vi "Measurement Logic.vi"() -> ()   [LabVIEW 2021, in "Quiescent Current_PMIC.lvlib"]
uses:
  Quiescent Current_PMIC.lvlib
  <instrlib>/niDCPower/nidcpower.llb/niDCPower Source Mode.ctl
  <instrlib>/niDCPower/nidcpower.llb/niDCPower Wait For Event - Event.ctl
  <instrlib>/niDCPower/nidcpower.llb/niDCPower Get Channel Name From String.vi
  <instrlib>/niDCPower/nidcpower.llb/niDCPower Output Function.ctl
  <instrlib>/niDCPower/nidcpower.llb/niDCPower Sequence Attribute Type.ctl
  <instrlib>/niDCPower/nidcpower.llb/niDCPower Create Advanced Sequence Step With Channels.vi
  Measurement Results.ctl
  <vilib>/Plug-In SDKs/Measurements/Measure Call Context/Measure Call Context.lvclass
  Measurement Configuration.ctl
panel:
  out "measurement results":T1
  in  "measurement configuration":T2={"DUT setup time"=1.0, "Source delay"=0.005, "Aperture time"=0.005, "Source resource name"="", "Source sense"=0, "Source current limit"=25.0, "Source maximum power"=300.0, "Source start voltage"=6.0, "Source stop voltage"=20.0, "Source voltage sweep points"=10} {"Source sense" items=["Local"=1008, "Remote"=1009]}
  out "measure call context out":refnum<class "Measure Call Context.lvclass">
  in  "measure call context in":refnum<class "Measure Call Context.lvclass">
  out "error out":errorcluster
  in  "error in":errorcluster
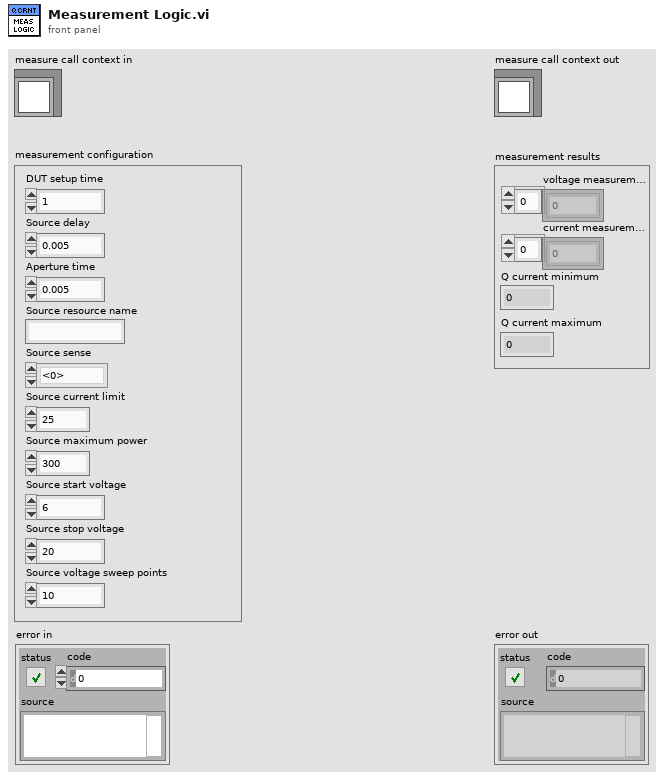
[diagram p1: front panel]
types:
  T1 = typedef "Quiescent Current_PMIC.lvlib/Measurement Results.ctl" = cluster{"Source voltages":dbl[], "Q currents":dbl[], "Q current minimum":dbl, "Q current maximum":dbl}
  T2 = typedef "Quiescent Current_PMIC.lvlib/Measurement Configuration.ctl" = cluster{"DUT setup time":dbl, "Source delay":dbl, "Aperture time":dbl, "Source resource name":string, "Source sense":i32, "Source current limit":dbl, "Source maximum power":dbl, "Source start voltage":dbl, "Source stop voltage":dbl, "Source voltage sweep points":i32}
  T3 = typedef "niDCPower Wait For Event - Event.ctl" = i32
  T4 = typedef "niDCPower Sequence Attribute Type.ctl" = i32
  T5 = typedef "niDCPower Output Function.ctl" = i32
  T6 = typedef "niDCPower Source Mode.ctl" = i32
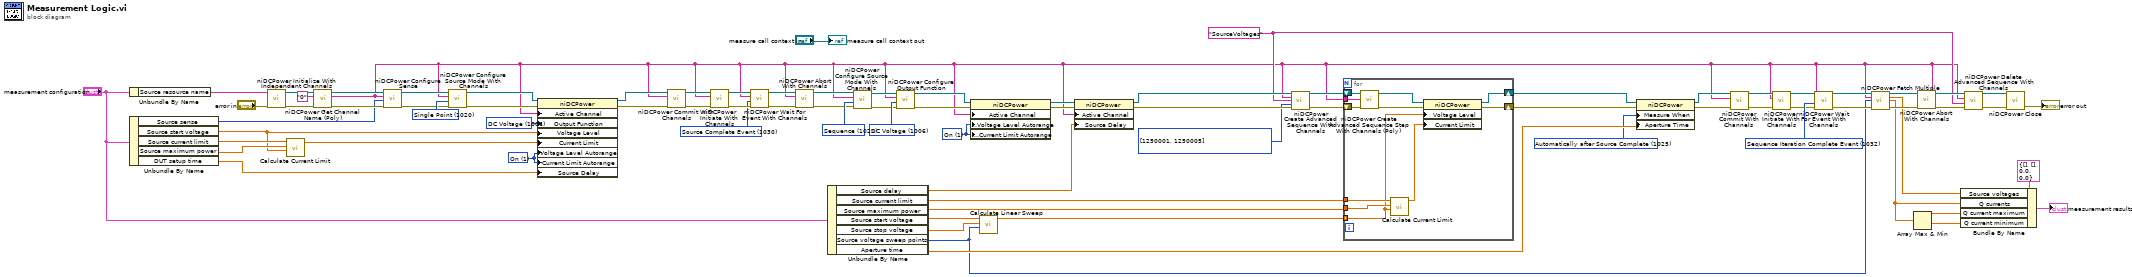
[diagram p0: block diagram]
diagram:
  w26 = T3 1032 items=["Source Complete Event"=1030, "Measure Complete Event"=1031, "Sequence Iteration Complete Event"=1032, "Sequence Engine Done Event"=1033] ("event")
  w40 = 1025 items=["Automatically after Source Complete"=1025, "On Demand"=1026, "On Measure Trigger"=1027] ("Measurement:Advanced:Measure When")
  w48 = 1 items=["Off", "On"] ("DC Voltage:Voltage Level Autorange")
  w47 = T4[] [1250001, 1250005] items=["Source -> Output Function"=1150008, "Source -> Output Enabled"=1250006, "Source -> Output Resistance"=1150061, "Source -> Transient Response"=1150062, "Source -> Custom Transient Response -> Voltage Gain Bandwidth"=1150067, "Source -> Custom Transient Response -> Voltage Compensation Frequency"=1150068, "Source -> Custom Transient Response -> Voltage Pole-Zero Ratio"=1150069, "Source -> Custom Transient Response -> Current Gain Bandwidth"=1150070, "Source -> Custom Transient Response -> Current Compensation Frequency"=1150071, "Source -> Custom Transient Response -> Current Pole-Zero Ratio"=1150072, "Source -> DC Voltage -> Voltage Level"=1250001, "Source -> DC Voltage -> Voltage Level Range"=1150005, "Source -> DC Voltage -> Current Limit"=1250005, "Source -> DC Voltage -> Current Limit High"=1150187, "Source -> DC Voltage -> Current Limit Low"=1150188, "Source -> DC Voltage -> Current Limit Range"=1150004, "Source -> DC Current -> Current Level"=1150009, "Source -> DC Current -> Current Level Range"=1150011, "Source -> DC Current -> Voltage Limit"=1150010, "Source -> DC Current -> Voltage Limit High"=1150185, "Source -> DC Current -> Voltage Limit Low"=1150186, "Source -> DC Current -> Voltage Limit Range"=1150012, "Source -> Pulse Voltage -> Pulse Voltage Level"=1150080, "Source -> Pulse Voltage -> Pulse Bias Voltage Level"=1150082, "Source -> Pulse Voltage -> Pulse Voltage Level Range"=1150084, "Source -> Pulse Voltage -> Pulse Current Limit"=1150081, "Source -> Pulse Voltage -> Pulse Current Limit High"=1150193, "Source -> Pulse Voltage -> Pulse Current Limit Low"=1150194, "Source -> Pulse Voltage -> Pulse Bias Current Limit"=1150083, "Source -> Pulse Voltage -> Pulse Bias Current Limit High"=1150195, "Source -> Pulse Voltage -> Pulse Bias Current Limit Low"=1150196, "Source -> Pulse Voltage -> Pulse Current Limit Range"=1150085, "Source -> Pulse Current -> Pulse Current Level"=1150086, "Source -> Pulse Current -> Pulse Bias Current Level"=1150088, "Source -> Pulse Current -> Pulse Current Level Range"=1150090, "Source -> Pulse Current -> Pulse Voltage Limit"=1150087, "Source -> Pulse Current -> Pulse Voltage Limit High"=1150189, "Source -> Pulse Current -> Pulse Voltage Limit Low"=1150190, "Source -> Pulse Current -> Pulse Bias Voltage Limit"=1150089, "Source -> Pulse Current -> Pulse Bias Voltage Limit High"=1150191, "Source -> Pulse Current -> Pulse Bias Voltage Limit Low"=1150192, "Source -> Pulse Current -> Pulse Voltage Limit Range"=1150091, "Source -> Advanced -> Source Delay"=1150051, "Source -> Advanced -> Pulse Bias Delay"=1150092, "Source -> Advanced -> Pulse On Time"=1150093, "Source -> Advanced -> Pulse Off Time"=1150094, "Source -> Advanced -> OVP Enabled"=1250002, "Source -> Advanced -> OVP Limit"=1250003, "Source -> Advanced -> Compliance Limit Symmetry"=1150184, "Source -> Advanced -> Sequence Step Delta Time"=1150198, "Measurement -> Sense"=1150013, "Measurement -> Aperture Time"=1150058, "Measurement -> Measure Record Length"=1150063, "Measurement -> Advanced -> DC Noise Rejection"=1150066, "Measurement -> Autorange"=1150244, "Measurement -> Advanced -> Autorange Behavior"=1150245, "Measurement -> Advanced -> Autorange Aperture Time Mode"=1150246, "Measurement -> Advanced -> Autorange Minimum Aperture Time"=1150247, "Measurement -> Advanced -> Autorange Minimum Aperture Time Units"=1150248, "Measurement -> Advanced -> Autorange Minimum Current Range"=1150255, "Measurement -> Advanced -> Autorange Minimum Voltage Range"=1150256, "Measurement -> Advanced -> Autorange Threshold Mode"=1150257, "Measurement -> Advanced -> Autorange Maximum Delay After Range Change"=1150322, "LCR -> Instrument Mode"=1150208, "LCR -> LCR Stimulus Function"=1150209, "LCR -> LCR Frequency"=1150210, "LCR -> LCR Voltage Amplitude"=1150211, "LCR -> LCR Current Amplitude"=1150212, "LCR -> LCR DC Bias Source"=1150213, "LCR -> LCR DC Bias Voltage Level"=1150214, "LCR -> LCR DC Bias Current Level"=1150215, "LCR -> LCR Impedance Autorange"=1150216, "LCR -> LCR Impedance Range"=1150217, "LCR -> LCR Measurement Time"=1150218, "LCR -> LCR Custom Measurement Time"=1150258, "LCR -> LCR Source Delay Mode"=1150315, "LCR -> Compensation -> Open -> Enabled"=1150220, "LCR -> Compensation -> Open -> Conductance"=1150261, "LCR -> Compensation -> Open -> Susceptance"=1150262, "LCR -> Compensation -> Short -> Enabled"=1150221, "LCR -> Compensation -> Short -> Resistance"=1150263, "LCR -> Compensation -> Short -> Reactance"=1150264, "LCR -> Compensation -> Load -> Enabled"=1150222, "LCR -> Compensation -> Load -> Measured Resistance"=1150268, "LCR -> Compensation -> Load -> Measured Reactance"=1150269, "LCR -> Compensation -> Load -> Actual Resistance"=1150270, "LCR -> Compensation -> Load -> Actual Reactance"=1150271] ("advanced sequence properties")
  w17 = "SourceVoltages" ("sequence name")
  w44 = T5 1006 items=["DC Voltage"=1006, "DC Current"=1007, "Pulse Voltage"=1049, "Pulse Current"=1050] ("output function")
  w43 = T6 1021 items=["Single Point"=1020, "Sequence"=1021] ("source mode")
  w65 = 1 items=["Off", "On"] ("Source:DC Voltage:Voltage Level Autorange")
  w66 = T3 1030 items=["Source Complete Event"=1030, "Measure Complete Event"=1031, "Sequence Iteration Complete Event"=1032, "Sequence Engine Done Event"=1033, "Pulse Complete Event"=1051, "Ready For Pulse Trigger Event"=1052] ("event")
  w77 = T6 1020 items=["Single Point"=1020, "Sequence"=1021] ("source mode")
  w72 = 1006 items=["DC Voltage"=1006, "DC Current"=1007, "Pulse Voltage"=1049, "Pulse Current"=1050] ("Source:Output Function")
  n1 = Unbundle By Name("measurement configuration") -> ("Source resource name"=w60:string)
  n2 = Unbundle By Name("measurement configuration") -> ("Source sense"=w1:i32, "Source start voltage"=w14:dbl, "Source current limit"=w32:dbl, "Source maximum power"=w31:dbl, "DUT setup time"=w64:dbl)
  n3 = call <instrlib>:"niDCPower Initialize With Independent Channels.vi"("error in (no error)"="error in", "resource name"=w60) -> ("error out"=w62:errorcluster, "instrument handle out"=w67:refnum<k15>)  [unwired: 8 in]
  n4 = call "Calculate Current Limit.vi"("Voltage value"=w14, "Maximum power"=w31, "Current limit in"=w32) -> ("Current limit out"=w30:dbl)  [unwired: 8 in]
  n5 = call-poly <instrlib>:"niDCPower Get Channel Name (Poly).vi"("error in (no error)"=w62, "index"="0", "instrument handle"=w67) -> ("error out"=w61:errorcluster, "name"=w2:string, "instrument handle out"=w63:refnum<k15>)  [unwired: 6 in]
  n6 = call <instrlib>:"niDCPower Configure Sense.vi"("error in (no error)"=w61, "sense"=w1, "channel name"=w2, "instrument handle"=w63) -> ("error out"=w75:errorcluster, "instrument handle out"=w73:refnum<k15>)  [unwired: 6 in]
  n7 = call <instrlib>:"niDCPower Configure Source Mode With Channels.vi"("error in (no error)"=w75, "source mode"=w77, "channel name"=w2, "instrument handle"=w73) -> ("error out"=w76:errorcluster, "instrument handle out"=w74:refnum<k15>)  [unwired: 6 in]
  n8 = property class="niDCPower"(reference=w74, error in=w76, "Active Channel"=w2, "Output Function"=w72, "Voltage Level"=w14, "Current Limit"=w30, "Voltage Level Autorange"=w65, "Current Limit Autorange"=w65, "Source Delay"=w64) -> (reference out=w78:refnum<k15>, error out=w79:errorcluster)
  n9 = call <instrlib>:"niDCPower Commit With Channels.vi"("error in (no error)"=w79, "channel name"=w2, "instrument handle"=w78) -> ("error out"=w81:errorcluster, "instrument handle out"=w80:refnum<k15>)  [unwired: 7 in]
  n10 = call <instrlib>:"niDCPower Initiate With Channels.vi"("error in (no error)"=w81, "channel name"=w2, "instrument handle"=w80) -> ("error out"=w68:errorcluster, "instrument handle out"=w69:refnum<k15>)  [unwired: 7 in]
  n11 = call <instrlib>:"niDCPower Wait For Event With Channels.vi"("error in (no error)"=w68, "event"=w66, "channel name"=w2, "instrument handle"=w69) -> ("error out"=w71:errorcluster, "instrument handle out"=w70:refnum<k15>)  [unwired: 6 in]
  n12 = call <instrlib>:"niDCPower Abort With Channels.vi"("error in (no error)"=w71, "channel name"=w2, "instrument handle"=w70) -> ("error out"=w34:errorcluster, "instrument handle out"=w35:refnum<k15>)  [unwired: 7 in]
  n13 = Unbundle By Name("measurement configuration") -> ("Source delay"=w58:dbl, "Source current limit"=w57:dbl, "Source maximum power"=w56:dbl, "Source start voltage"=w29:dbl, "Source stop voltage"=w27:dbl, "Source voltage sweep points"=w9:i32, "Aperture time"=w55:dbl)
  n14 = call <instrlib>:"niDCPower Configure Source Mode With Channels.vi"("error in (no error)"=w34, "source mode"=w43, "channel name"=w2, "instrument handle"=w35) -> ("error out"=w41:errorcluster, "instrument handle out"=w42:refnum<k15>)  [unwired: 6 in]
  n15 = call <instrlib>:"niDCPower Configure Output Function.vi"("error in (no error)"=w41, "output function"=w44, "channel name"=w2, "instrument handle"=w42) -> ("error out"=w52:errorcluster, "instrument handle out"=w51:refnum<k15>)  [unwired: 6 out]
  n16 = property class="niDCPower"(reference=w51, error in=w52, "Active Channel"=w2, "Source:DC Voltage:Voltage Level Autorange"=w48, "Source:DC Voltage:Current Limit Autorange"=w48) -> (reference out=w49:refnum<k15>, error out=w50:errorcluster)
  n17 = call "Calculate Linear Sweep.vi"("Points"=w9, "Stop level"=w27, "Start level"=w29) -> ("Values"=w28:dbl[])  [unwired: 8 in]
  n18 = property class="niDCPower"(reference=w49, error in=w50, "Active Channel"=w2, "Source Delay"=w58) -> (reference out=w53:refnum<k15>, error out=w54:errorcluster)
  n19 = call <instrlib>:"niDCPower Create Advanced Sequence With Channels.vi"("instrument handle"=w53, "channel name"=w2, "sequence name"=w17, "advanced sequence properties"=w47, "error in (no error)"=w54) -> ("instrument handle out"=w45:refnum<k15>, "error out"=w46:errorcluster)  [unwired: 9 in]
  n20 = for {
    shift-right: [w90] -> w36
    shift-left: w46 -> [w93]
    shift-right: [w83] -> w37
    shift-left: w45 -> [w89]
    tunnel: w56 -> [w86]
    tunnel: w28 -> [w85] mode=indexing
    tunnel: w57 -> [w87]
    tunnel: w2 -> [w88]
    n21 = call-poly <instrlib>:"niDCPower Create Advanced Sequence Step With Channels (Poly).vi"("error in (no error)"=w93, "channel name"=w88, "instrument handle"=w89) -> ("error out"=w91:errorcluster, "instrument handle out"=w92:refnum<k15>)  [unwired: 7 in]
    n22 = call "Calculate Current Limit.vi"("Voltage value"=w85, "Maximum power"=w86, "Current limit in"=w87) -> ("Current limit out"=w84:dbl)  [unwired: 8 in]
    n23 = property class="niDCPower"(reference=w92, error in=w91, "Voltage Level"=w85, "Current Limit"=w84) -> (reference out=w83:refnum<k15>, error out=w90:errorcluster)
  }
  n24 = property class="niDCPower"(reference=w37, error in=w36, "Measure When"=w40, "Aperture Time"=w55) -> (reference out=w38:refnum<k15>, error out=w39:errorcluster)
  n25 = call <instrlib>:"niDCPower Commit With Channels.vi"("error in (no error)"=w39, "channel name"=w2, "instrument handle"=w38) -> ("error out"=w25:errorcluster, "instrument handle out"=w23:refnum<k15>)  [unwired: 7 in]
  n26 = call <instrlib>:"niDCPower Initiate With Channels.vi"("error in (no error)"=w25, "channel name"=w2, "instrument handle"=w23) -> ("error out"=w24:errorcluster, "instrument handle out"=w22:refnum<k15>)  [unwired: 7 in]
  n27 = call <instrlib>:"niDCPower Wait For Event With Channels.vi"("error in (no error)"=w24, "event"=w26, "channel name"=w2, "instrument handle"=w22) -> ("error out"=w13:errorcluster, "instrument handle out"=w11:refnum<k15>)  [unwired: 6 in]
  n28 = call <instrlib>:"niDCPower Fetch Multiple.vi"("instrument handle"=w11, "channel name"=w2, "count (1)"=w9, "error in (no error)"=w13) -> ("instrument handle out"=w10:refnum<k15>, "voltage measurements"=w6:dbl[], "current measurements"=w5:dbl[], "error out"=w12:errorcluster)  [unwired: 1 in, 7 out]
  n29 = Array Max & Min(array=w5) -> (max value=w4:dbl, min value=w3:dbl)  [unwired: 2 out]
  n30 = call <instrlib>:"niDCPower Abort With Channels.vi"("error in (no error)"=w12, "channel name"=w2, "instrument handle"=w10) -> ("error out"=w20:errorcluster, "instrument handle out"=w19:refnum<k15>)  [unwired: 7 in]
  n31 = Bundle By Name(cluster=T1 {"Source voltages"=[], "Q currents"=[], "Q current minimum"=0.0, "Q current maximum"=0.0} ("measurement results"), "Source voltages"=w6, "Q currents"=w5, "Q current maximum"=w4, "Q current minimum"=w3) -> (→"measurement results":T1)
  n32 = call <instrlib>:"niDCPower Delete Advanced Sequence With Channels.vi"("error in (no error)"=w20, "sequence name"=w17, "channel name"=w2, "instrument handle"=w19) -> ("error out"=w21:errorcluster, "instrument handle out"=w18:refnum<k15>)  [unwired: 6 in]
  n33 = call <instrlib>:"niDCPower Close.vi"("error in (no error)"=w21, "instrument handle"=w18) -> ("error out"=→"error out":errorcluster)  [unwired: 9 in]
  "measure call context out" <- "measure call context in"
